vi "Reset Laser Power.vi"(8 "error in (no error)":errorcluster, 10 "Shutter Enable":bool[](array[boolean]), 11 "Application in":refnum<class "Application.lvclass">) -> (0 "error out":errorcluster, 3 "Application out":refnum<class "Application.lvclass">)   [LabVIEW 2018, in "Application.lvlib" / "Application.lvclass"]
uses:
  Application.lvclass
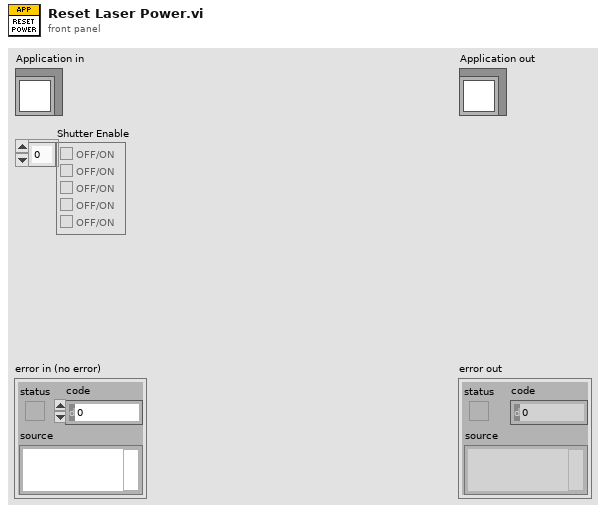
[diagram p1: front panel]
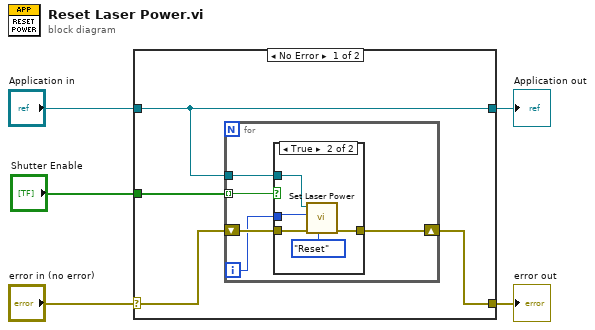
[diagram p0: block diagram]
diagram:
  n1 = case shown="No Error" "error in (no error)" {
    selector: "error in (no error)" -> [w9 w22]
    tunnel: [w8 w22] -> w4
    tunnel: [w6 w21] -> w2
    tunnel: "Application in" -> [w6 w21]
    tunnel: "Shutter Enable" -> [w7 _]
    frame No Error {
      n2 = for {
        shift-right: [w13] -> w8
        shift-left: w9 -> [w14]
        tunnel: w7 -> [w12] mode=indexing
        tunnel: w6 -> [w10]
        i -> [w11]
        n3 = case shown="True" w12 {
          tunnel: w14 -> [w15 w20]
          tunnel: [w15 w19] -> w13
          tunnel: w11 -> [_ w18]
          tunnel: w10 -> [_ w17]
          frame False {
          }
          frame True {
            n4 = call-dynamic "Set Laser Power.vi"("Mode"=enum16{"Normal", "Ignore", "Reset"}."Reset", "error in (no error)"=w20, "laser index"=w18, "Application in"=w17) -> ("error out"=w19:errorcluster)  [unwired: 6 in, 1 out]
          }
        }
      }
    }
    frame Error {
    }
  }
  "error out" <- w4
  "Application out" <- w2
